vi "myRIO Support.vi"(8 "Error In":errorcluster) -> (0 "Error Out":errorcluster)   [LabVIEW 2011, in "LVH-LINX.lvlib"]
doc: "NI myRIO is only supported by LabVIEW 2013 and later. \n\nIn order to provide LINX support for LabVIEW 2011 and 2012 all NI myRIO support is disabled by default. \n\n If you are using LabVIEW 2013 or later and have the NI myRIO module installed you can use this wizard \nto enable LINX myRIO support."
uses:
  vi.lib/LabVIEW Hacker/LINX/LVH-LINX.lvlib
  <vilib>/Utility/traverseref.llb/TRef TravTarget.ctl
  <vilib>/Utility/traverseref.llb/VI Scripting - Traverse.lvlib
  <vilib>/LabVIEW Hacker/LVH-Toolbox/Common/LVH-Common.lvlib
panel:
  out "Status":string
  out "Slide":u8(slide) scale=0.0..100.0
  in  "Finish":bool
  in  "Disable":bool
  in  "Enable":bool
  # "NI myRIO is only supported by LabVIEW 2013 and later.  \n\nIn order to provide LINX support for LabVIEW 2011 and 2012 all NI myRIO support is disabled by default. \n\nIf you are using LabVIEW 2013 or later and have the NI myRIO module installed you can use this wizard \nto enable LINX myRIO support."
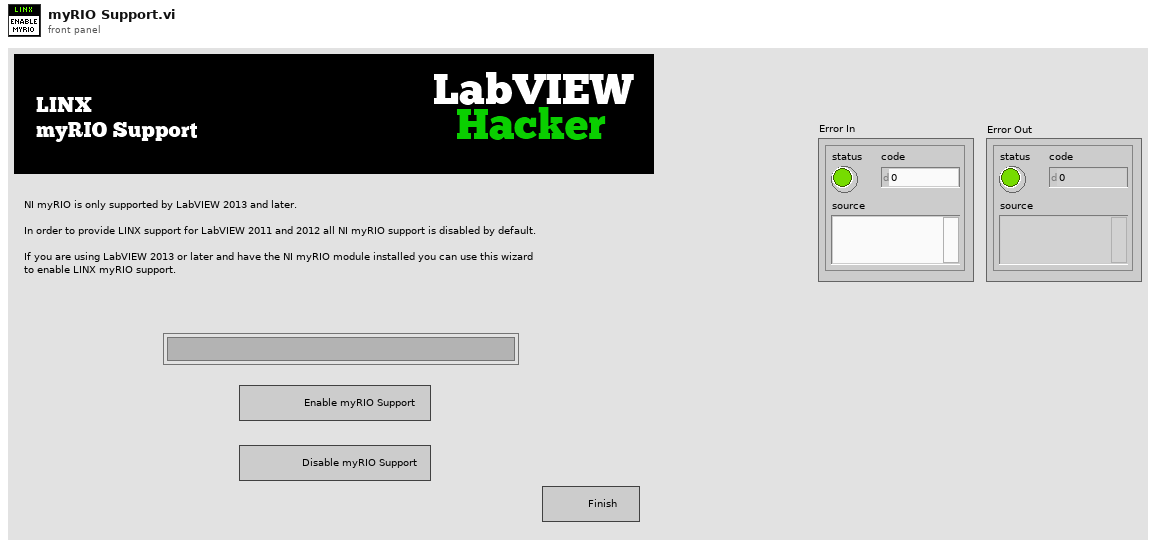
[diagram p1: front panel]
types:
  T1 = enum8{"Enabled", "Disabled", "Disabled and Grayed Out"}
  T2 = typedef "TRef TravTarget.ctl" = enum16{"FP", "BD", "Other"}
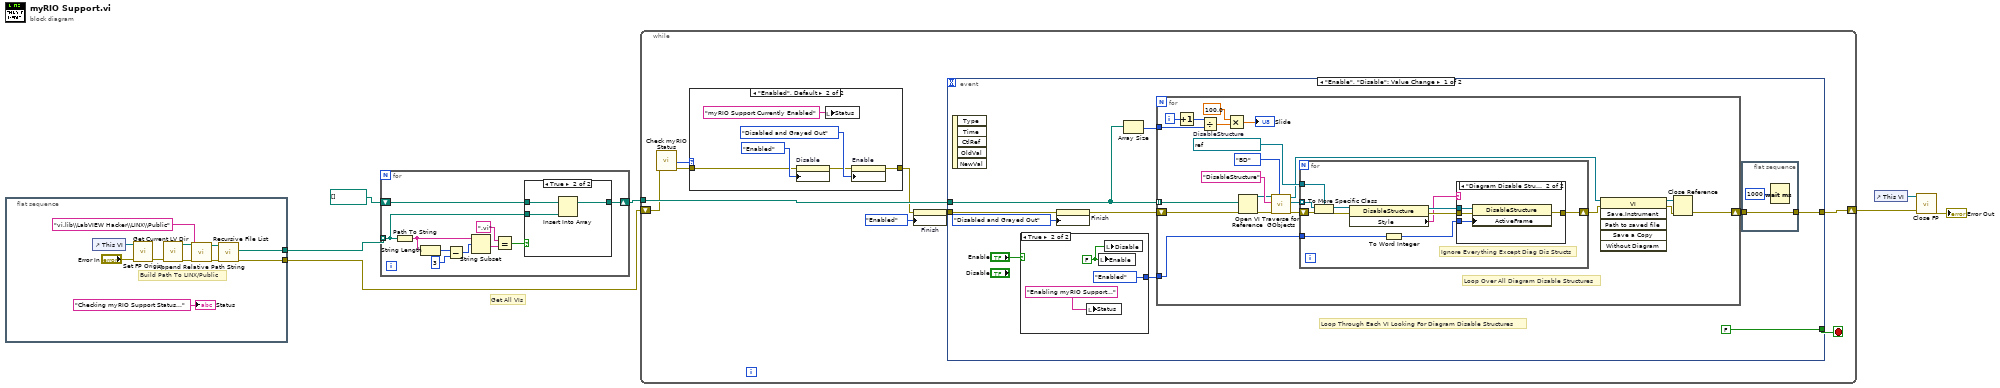
[diagram p0: block diagram]
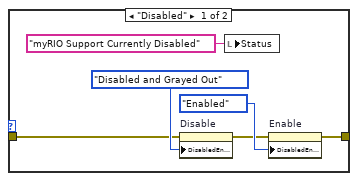
[diagram p2: hidden frame]
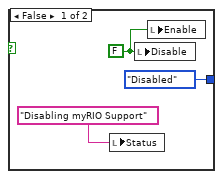
[diagram p3: hidden frame]
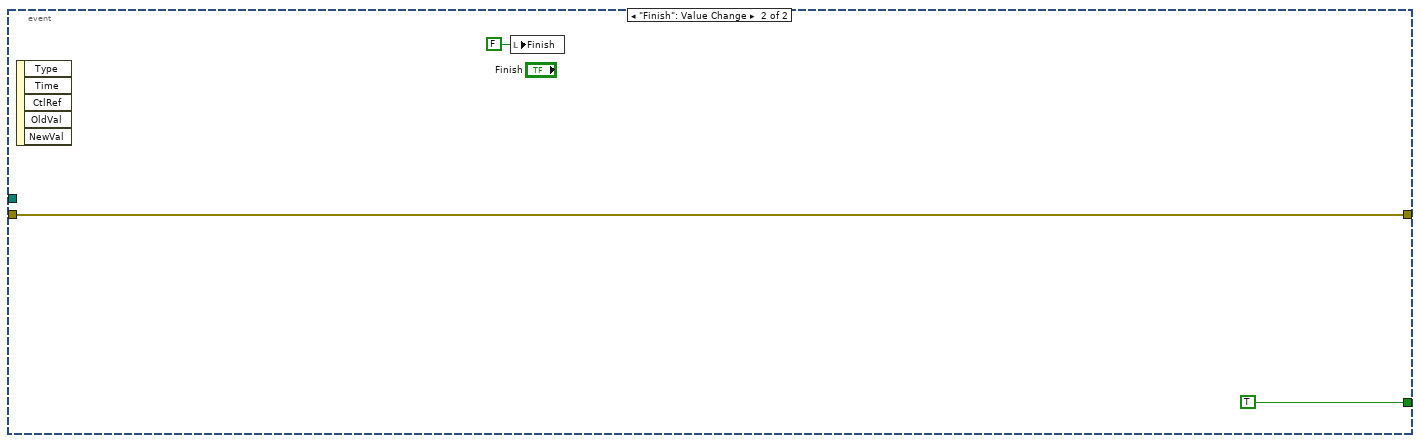
[diagram p5: hidden frame]
diagram:
  # "Get All VIs"
  n1 = flat-sequence {
    tunnel: [w18] -> w6
    tunnel: [w17] -> w4
    frame #0 {
      # "Build Path To LINX/Public"
      n2 = control-ref of="This VI"() -> (w12:refnum<vi>)
      n3 = call <vilib>:"Set FP Origin.vi"("Error In"="Error In", "VI Ref"=w12) -> ("Error Out"=w11:errorcluster)  [unwired: 9 in]
      n4 = call <vilib>:"Get Current LV Dir.vi"("Error In"=w11) -> ("Error Out"=w15:errorcluster, "This LV Directory"=w16:path)  [unwired: 9 in]
      n5 = call <vilib>:"Append Relative Path String.vi"("Error In"=w15, "Relative Path"="vi.lib\\LabVIEW Hacker\\LINX\\Public", "Base Path"=w16) -> ("Error Out"=w13:errorcluster, "Absolute Path"=w9:path)  [unwired: 7 in]
      n6 = call <vilib>:"Recursive File List.vi"("error in (no error)"=w13, "Folder Path"=w9) -> ("error out"=w17:errorcluster, "All Files in Dir"=w18:path[])  [unwired: 5 in, 3 out]
      "Status" <- "Checking myRIO Support Status..." ("Status")
    }
  }
  n7 = for {
    tunnel: w6 -> [w26] mode=indexing
    shift-right: [w27] -> w5
    shift-left: path[] [] ("array") -> [w28]
    n8 = Path To String(path=w26) -> (string=w25:string)
    n9 = String Length(string=w25) -> (length=w24:i32)
    n10 = Subtract(x=w24, y=3) -> (x-y=w22:i32)
    n11 = String Subset(string=w25, offset (0)=w22) -> (substring=w21:string)  [unwired: 1 in]
    n12 = Equal?(x=".vi", y=w21) -> (x = y?=w19:bool)
    n13 = case shown="True" w19 {
      tunnel: w26 -> [_ w32]
      tunnel: w28 -> [w29 w31]
      tunnel: [w29 w30] -> w27
      frame False {
      }
      frame True {
        n14 = Insert Into Array(array=w31, new element=w32) -> (w30:path[])  [unwired: 1 in]
      }
    }
  }
  n15 = while {
    tunnel: w5 -> [w41]
    shift-right: [w39] -> w3
    shift-left: w4 -> [w36]
    stop <- w40 stop-if-true
    n16 = call "Check myRIO Status.vi"("Error In"=w36) -> ("Error Out"=w34:errorcluster, "myRIO Support Status"=w35:enum16{"Enabled", "Disabled"})  [unwired: 9 in]
    n17 = case shown="\"Enabled\", Default" w35 {
      tunnel: w34 -> [w45 w51]
      tunnel: [w43 w49] -> w33
      frame "Disabled" {
        n18 = property on="Disable" class="Bool (strict)"(error in=w45, "DisabledEnum"=T1."Disabled and Grayed Out" ("Disabled")) -> (error out=w44:errorcluster)  [unwired: 1 in, 1 out]
        n19 = local write "Status"("myRIO Support Currently Disabled" ("Status")) -> ()
        n20 = property on="Enable" class="Bool (strict)"(error in=w44, "DisabledEnum"=T1."Enabled" ("Disabled")) -> (error out=w43:errorcluster)  [unwired: 1 in, 1 out]
      }
      frame "Enabled", Default {
        n21 = property on="Disable" class="Bool (strict)"(error in=w51, "DisabledEnum"=T1."Enabled" ("Disabled")) -> (error out=w50:errorcluster)  [unwired: 1 in, 1 out]
        n22 = local write "Status"("myRIO Support Currently Enabled" ("Status")) -> ()
        n23 = property on="Enable" class="Bool (strict)"(error in=w50, "DisabledEnum"=T1."Disabled and Grayed Out" ("Disabled")) -> (error out=w49:errorcluster)  [unwired: 1 in, 1 out]
      }
    }
    n24 = property on="Finish" class="Bool (strict)"(error in=w33, "DisabledEnum"=T1."Enabled" ("Disabled")) -> (error out=w37:errorcluster)  [unwired: 1 in, 1 out]
    n25 = event shown="[0] \"Enable\", \"Disable\": Value Change" {
      selector: _ -> [_ _]
      dyn-events: _ -> [_ _]
      timeout: _ -> [_ _]
      tunnel: w41 -> [w60 _]
      tunnel: w37 -> [w56 w109]
      tunnel: [w54 w109] -> w39
      tunnel: [FALSE TRUE] -> w40
      event "Enable", "Disable": Value Change {
        # "Loop Through Each VI Looking For Diagram Disable Structures"
        n26 = event-data() -> ()  [unwired: 1 in, 5 out]
        n27 = case shown="True" "Enable" {
          tunnel: [enum16{"Enabled", "Disabled"}."Disabled" ("myRIO Support") enum16{"Enabled", "Disabled"}."Enabled" ("myRIO Support")] -> w63
          frame False {
            w66 = FALSE ("Disable")
            n28 = local write "Status"("Disabling myRIO Support" ("Status")) -> ()
            n29 = local write "Disable"(w66) -> ()
            n30 = local write "Enable"(w66) -> ()
          }
          frame True {
            w69 = FALSE ("Enable")
            n31 = local write "Status"("Enabling myRIO Support..." ("Status")) -> ()
            n32 = local write "Enable"(w69) -> ()
            n33 = local write "Disable"(w69) -> ()
          }
        }
        n34 = property on="Finish" class="Bool (strict)"(error in=w56, "DisabledEnum"=T1."Disabled and Grayed Out" ("Disabled")) -> (error out=w57:errorcluster)  [unwired: 1 in, 1 out]
        n35 = Array Size(array=w60) -> (size(s)=w59:i32)
        n36 = for {
          tunnel: w60 -> [w86] mode=indexing
          shift-right: [w83] -> w55
          shift-left: w57 -> [w85]
          tunnel: w63 -> [w78]
          tunnel: w59 -> [w77]
          i -> [w73]
          w90 = refnum<vi> refnum  # DisableStructure
          # "Loop Over All Diagram Disable Structures"
          n37 = Increment(x=w73) -> (x+1=w72:i32)
          n38 = Divide(x=w72, y=w77) -> (x/y=w76:dbl)
          n39 = Multiply(x=100.0, y=w76) -> (x*y=→"Slide":dbl)
          n40 = Open VI Reference(vi path=w86, error in (no error)=w85) -> (vi reference=w87:refnum<vi>, error out=w92:errorcluster)  [unwired: 4 in]
          n41 = call <vilib>:"Traverse for GObjects.vi"("Traverse Target"=TRef_TravTarget."BD", "error in (no error)"=w92, "Class Name"="DisableStructure", "VI Refnum"=w87) -> ("error out"=w91:errorcluster, "References"=w84:refnum<vi>[], "dup VI Refnum"=w80:refnum<vi>)  [unwired: 4 in, 1 out]
          n42 = for {
            tunnel: w90 -> [w102]
            tunnel: w84 -> [w101] mode=indexing
            shift-right: [w100] -> w79
            shift-left: w91 -> [w103]
            tunnel: w78 -> [w94]
            # "Ignore Everything Except Diag Dis Structs"
            n43 = To More Specific Class(target class=w102, reference=w101, error in=w103) -> (specific class reference=w97:refnum<vi>, error out=w99:errorcluster)
            n44 = property class="DisableStructure"(reference=w97, error in=w99) -> (reference out=w96:refnum<vi>, error out=w98:errorcluster, "Style"=w95:string)
            n45 = To Word Integer(number=w94) -> (16bit integer=w93:i16)
            n46 = case shown="\"Diagram Disable Structure\"" w95 {
              tunnel: w93 -> [_ w108]
              tunnel: [w104 w107] -> w100
              tunnel: w98 -> [w104 w106]
              tunnel: w96 -> [_ w105]
              frame Default {
              }
              frame "Diagram Disable Structure" {
                n47 = property class="DisableStructure"(reference=w105, error in=w106, "ActiveFrame"=w108) -> (error out=w107:errorcluster)  [unwired: 1 out]
              }
            }
          }
          n48 = invoke class="VI" method="Save.Instrument"(reference=w80, error in=w79) -> (reference out=w82:refnum<vi>, error out=w81:errorcluster)  [unwired: 4 in, 4 out]
          n49 = Close Reference(reference=w82, error in (no error)=w81) -> (error out=w83:errorcluster)
        }
        n50 = flat-sequence {
          tunnel: w55 -> [w65]
          tunnel: [w65] -> w54
          frame #0 {
            n51 = Wait (ms)(milliseconds to wait=u32 1000) -> ()  [unwired: 1 out]
          }
        }
      }
      event "Finish": Value Change {
        n52 = event-data() -> ()  [unwired: 1 in, 5 out]
        n53 = local write "Finish"(FALSE ("Finish")) -> ()
      }
    }
  }
  n54 = control-ref of="This VI"() -> (w1:refnum<vi>)
  n55 = call <vilib>:"Close FP.vi"("Error In"=w3, "VI Ref"=w1) -> ("Error Out"=→"Error Out":errorcluster)  [unwired: 9 in]
